vi "9614 Invalid Access Type--errror.vi"(8 "error in":errorcluster, 11 "Access Type":string) -> (0 "error out":errorcluster)   [LabVIEW 2024, in "Electronic Datasheet.lvlib"]
uses:
  Electronic Datasheet.lvlib
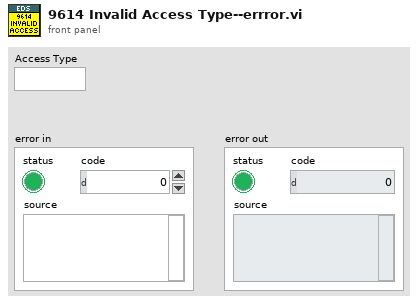
[diagram p1: front panel]
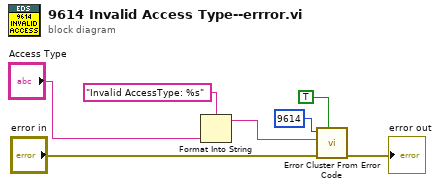
[diagram p0: block diagram]
diagram:
  n1 = Format Into String(format string="Invalid AccessType: %s" ("error message (\"\")"), "Access Type") -> (resulting string=w3:string)  [unwired: 2 in, 1 out]
  n2 = call <vilib>:"Error Cluster From Error Code.vi"("show call chain? (False)"=TRUE, "error in (no error)"="error in", "error message (\"\")"=w3, "error code (0)"=9614) -> ("error out"=→"error out":errorcluster)  [unwired: 5 in]
